vi "ORP电极校准.vi"() -> ()   [LabVIEW 2016, in "斯坦道多参数.lvlib"]
uses:
  <vilib>/Utility/miscctls.llb/LVPointTypeDef.ctl
  <vilib>/Analysis/NI_AALBase.lvlib
  <vilib>/Utility/config.llb/NI_LVConfig.lvlib
panel:
  out "滤波设定":dbl
  in  "刷新按钮":bool
  out "第二点信号值":dbl
  out "第一点信号值":dbl
  out "通讯状态":string
  out "温度":dbl format="%#.2f"
  out "当前信号值":dbl caption="信号值" format="%#.2f"
  in  "校准停止":bool
  in  "校准启动":bool
  out "波形图表":sgl(graph) caption="历史曲线"
  out "第二点校准值":dbl
  out "第一点校准值":dbl
  in  "校准模式":u16(ring) items=["单点校准"]
  out "提示":string
  out "最小值":sgl format="%#.2f"
  out "最大值":sgl format="%#.2f"
  out "mean":dbl caption="均值" format="%#.2f"
  out "standard deviation":dbl caption="标准差" format="%#.2f"
  out "变异系数":dbl format="%#.6f"
  in  "标液1":dbl
  out "当前读取值":dbl caption="测量值" format="%#.2f"
  out "ORP偏移修正值":dbl format="%#.2f"
  # "ORP电极设定"
  # "请选择校准模式:"
  # "℃"
  # "mV"
  # "mV"
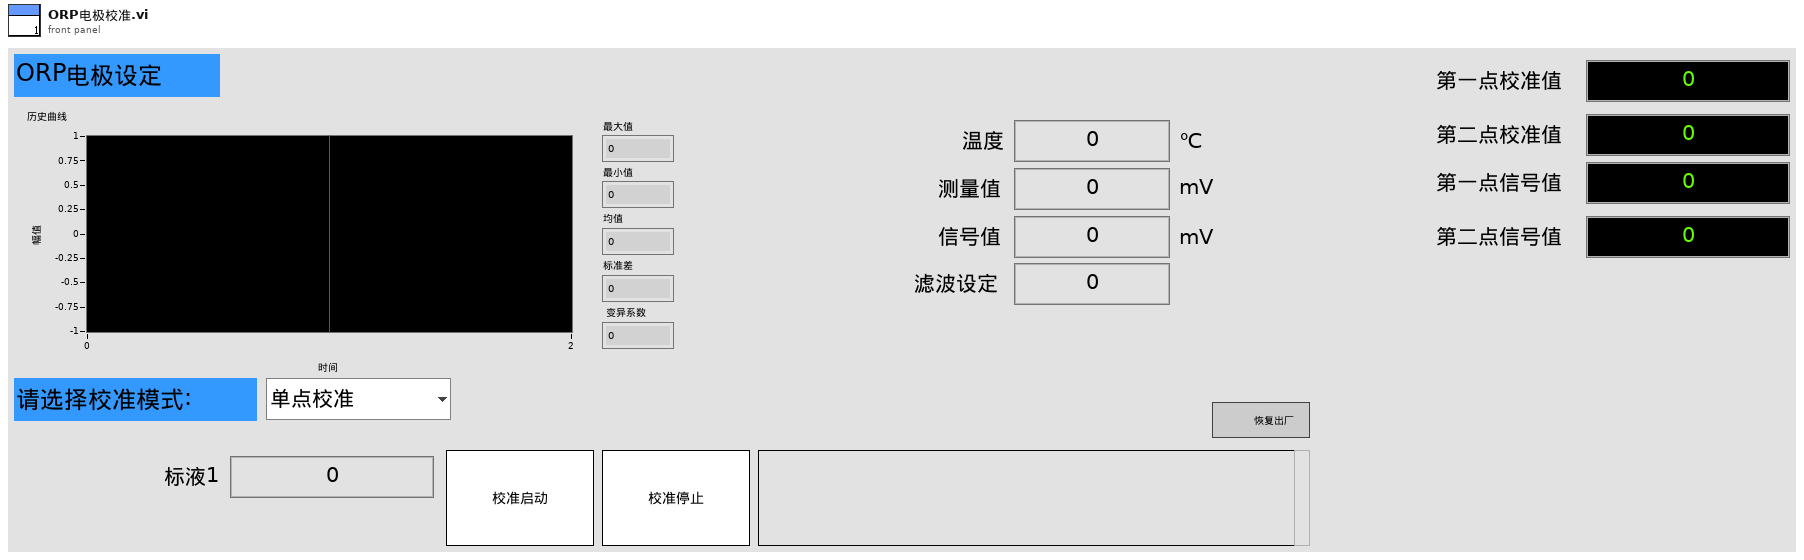
[diagram p1: front panel]
types:
  T1 = typedef "LVPointTypeDef.ctl" = cluster{"Horizontal":i16, "Vertical":i16}
  T2 = typedef "NI_LVConfig.lvlib/Config Data RefNum.ctl" = refnum<k1>
  T3 = cluster{"电极状态标志":u16, "电极型号标志":u16, "测量值":sgl, "温度测量值":sgl, "信号值":sgl, "温度信号值":sgl, "000AH_NC":sgl, "偏移修正值":sgl, "温度偏移修正值":sgl, "手动温度补偿值":sgl, "命令滤波设定":u16, "温度模式":enum16{"ATC", "MTC"}, "生产批次":u16, "传感器序号":u16, "串口地址":u16, "串口波特率":enum16{"9600", "19200", "115200"}, "串口校验位":enum16{"NONE", "ODD", "EVEN"}, "串口停止位":enum16{"1bit", "2bit"}}
  T4 = enum8{"Enabled", "Disabled", "Disabled and Grayed Out"}
  T5 = cluster{"ph":bool, "DO":bool, "Cond":bool, "Turb":bool, "叶绿素a":bool, "藻密度":bool, "ORP":bool}
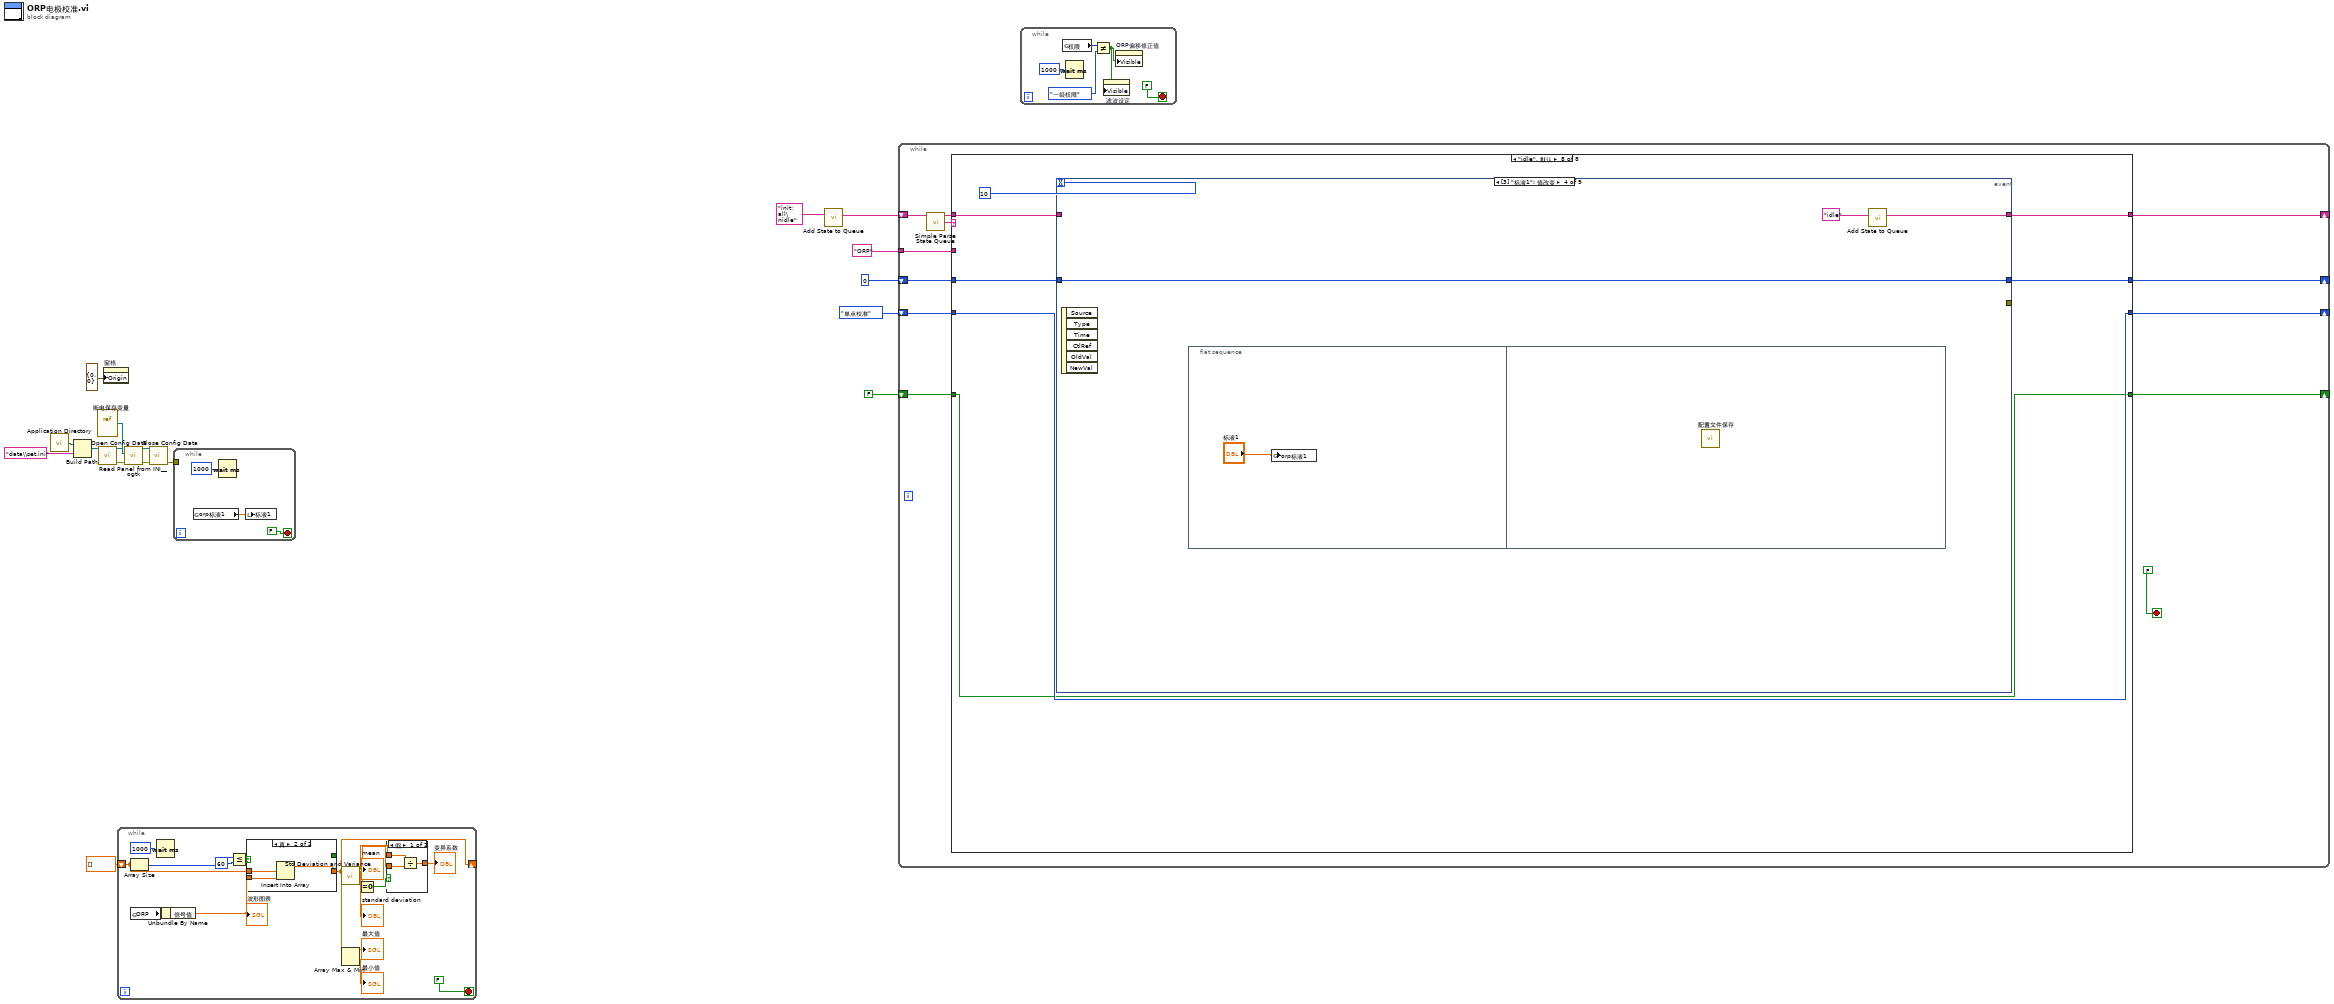
[diagram p0: block diagram]
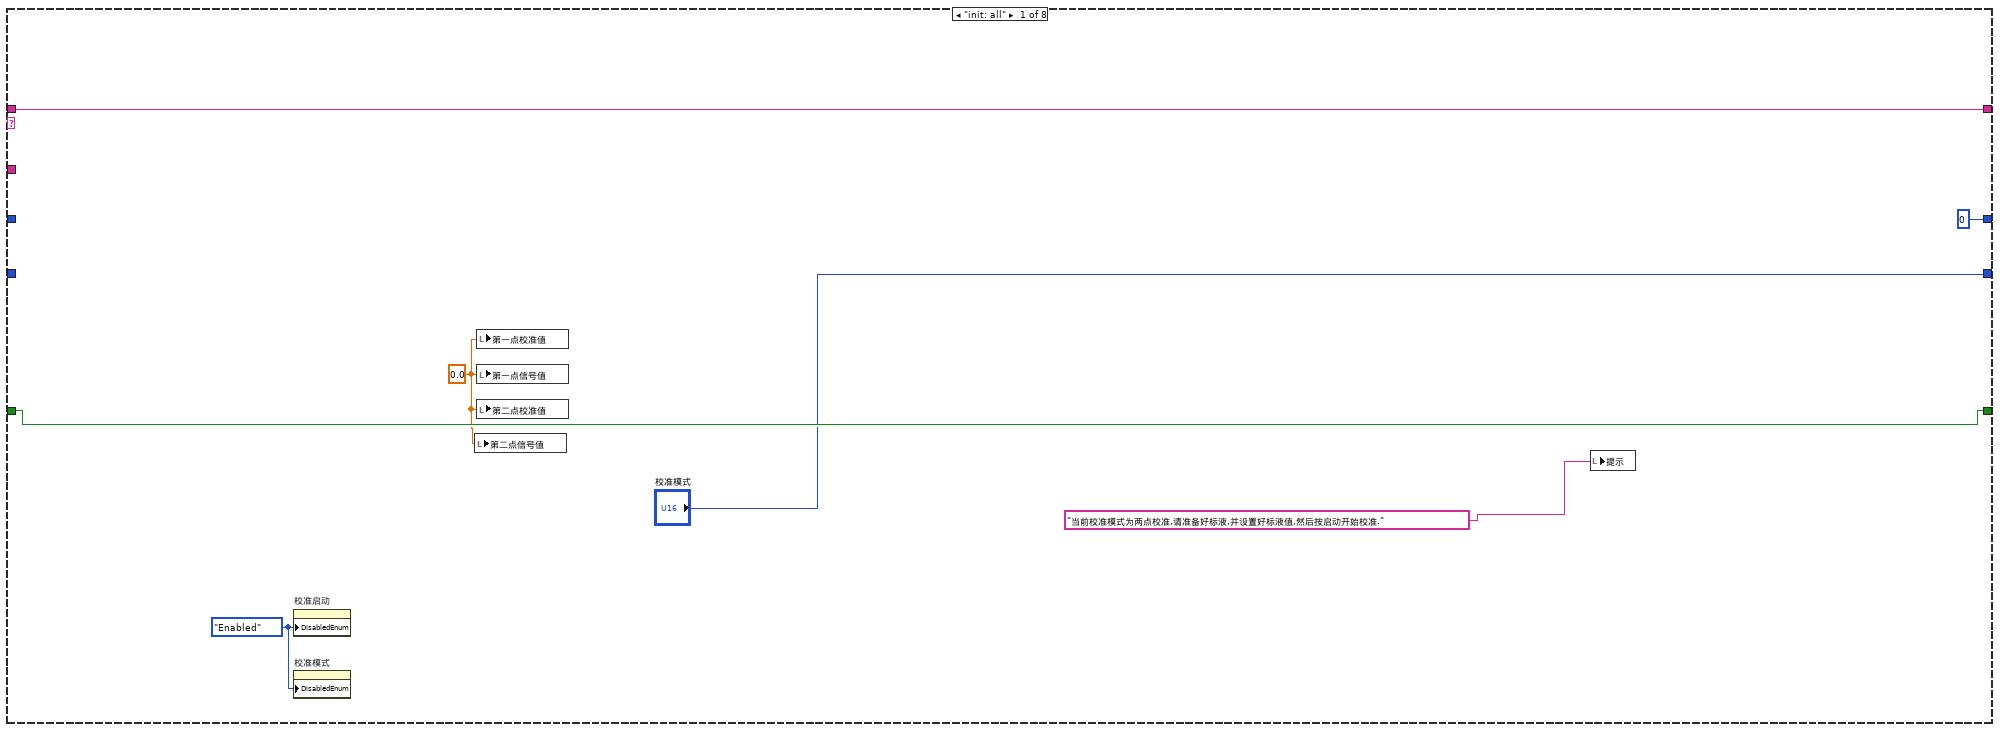
[diagram p2: hidden frame]
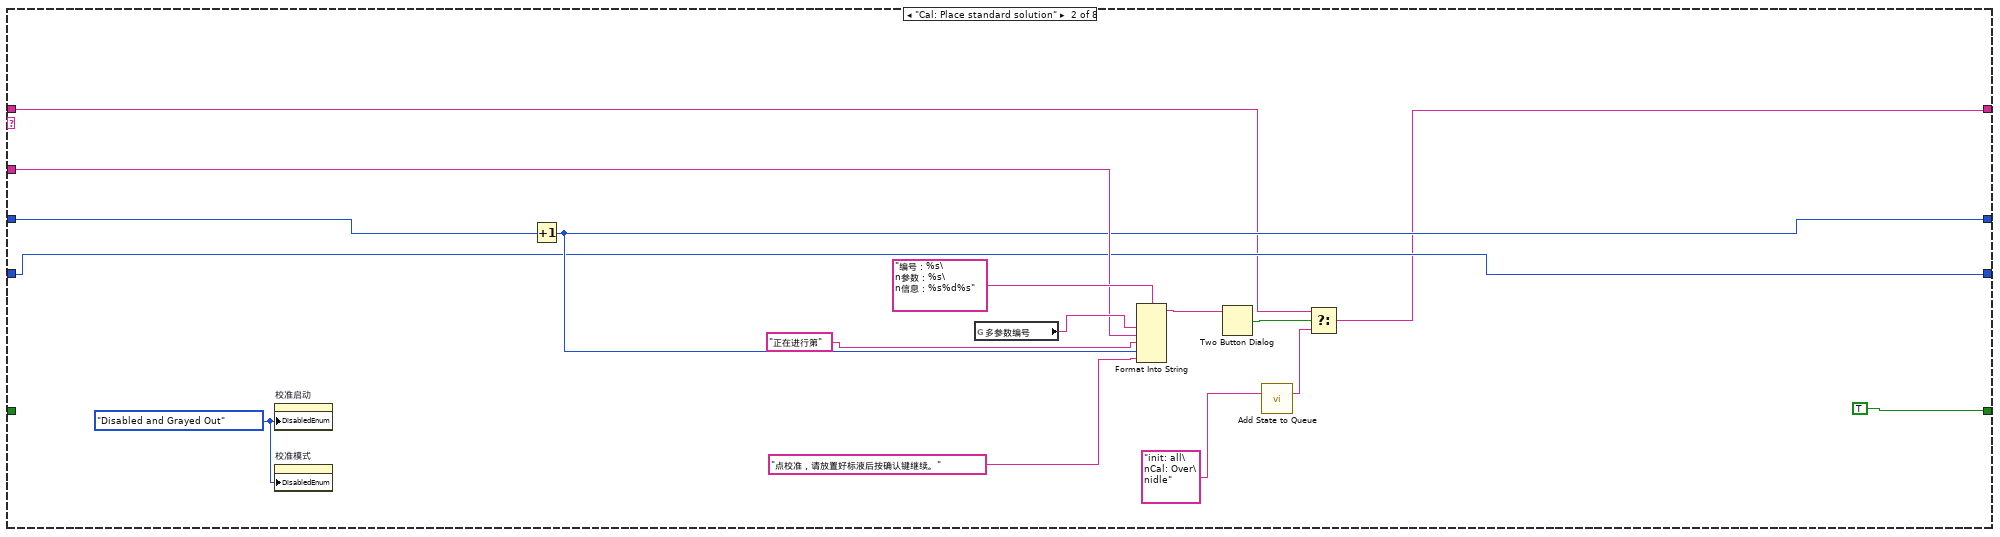
[diagram p3: hidden frame]
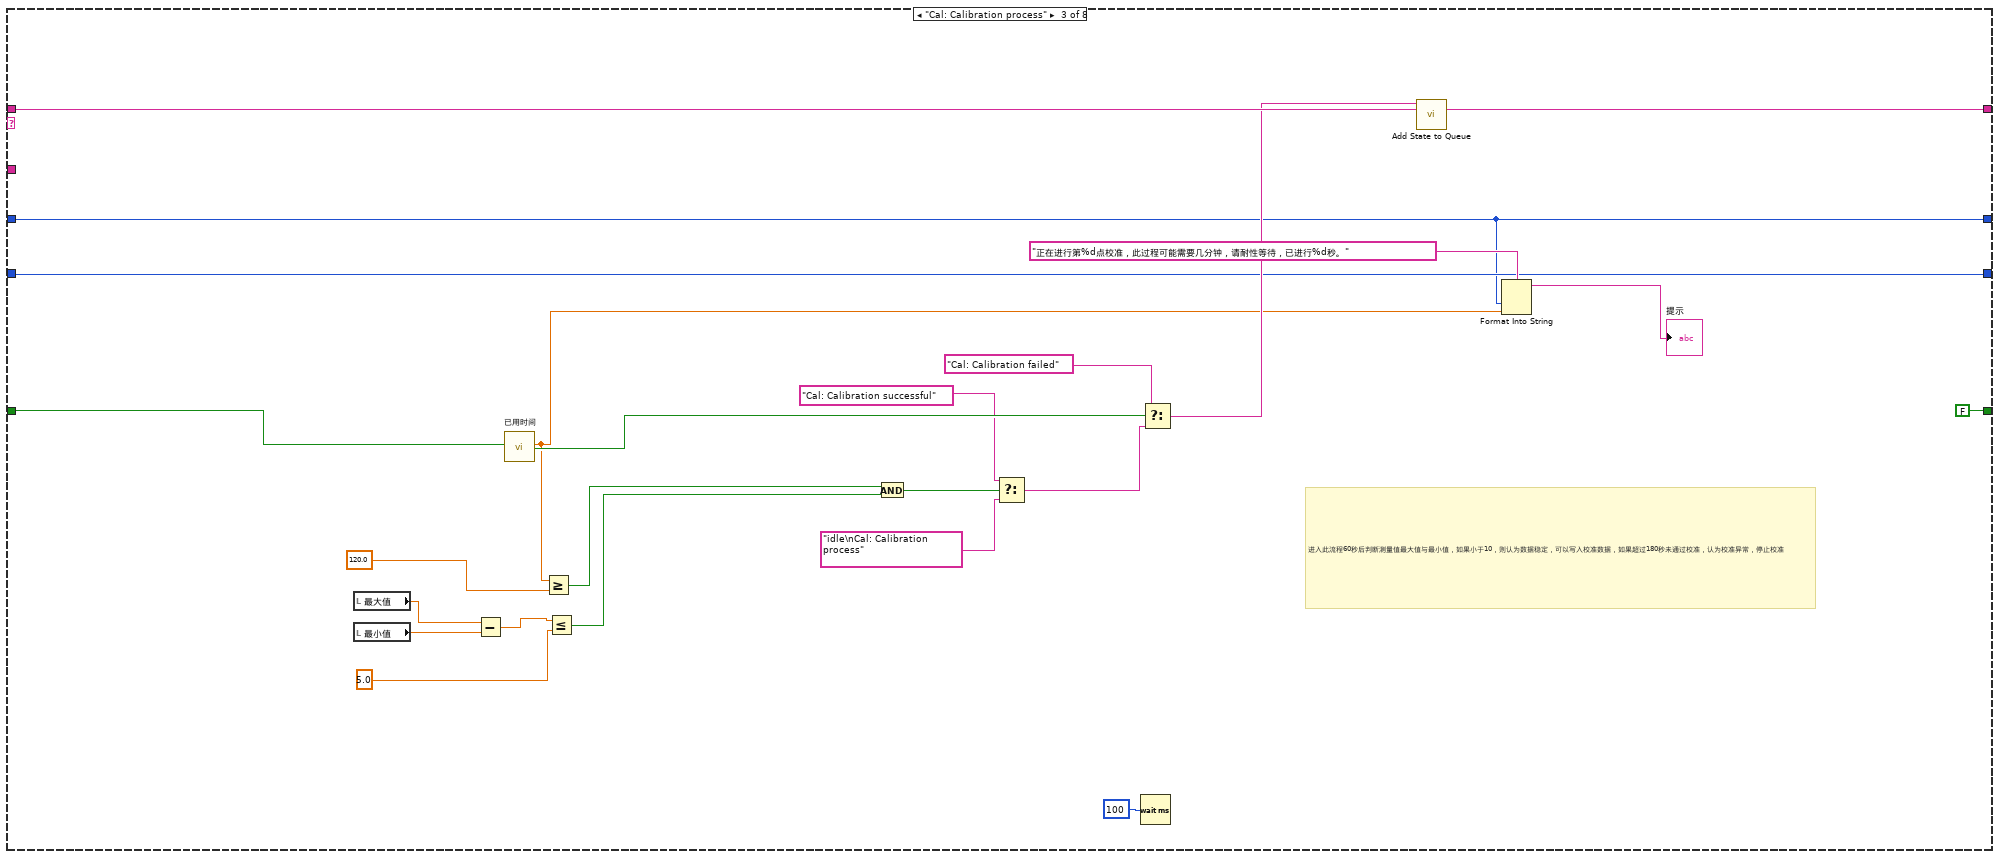
[diagram p4: hidden frame]
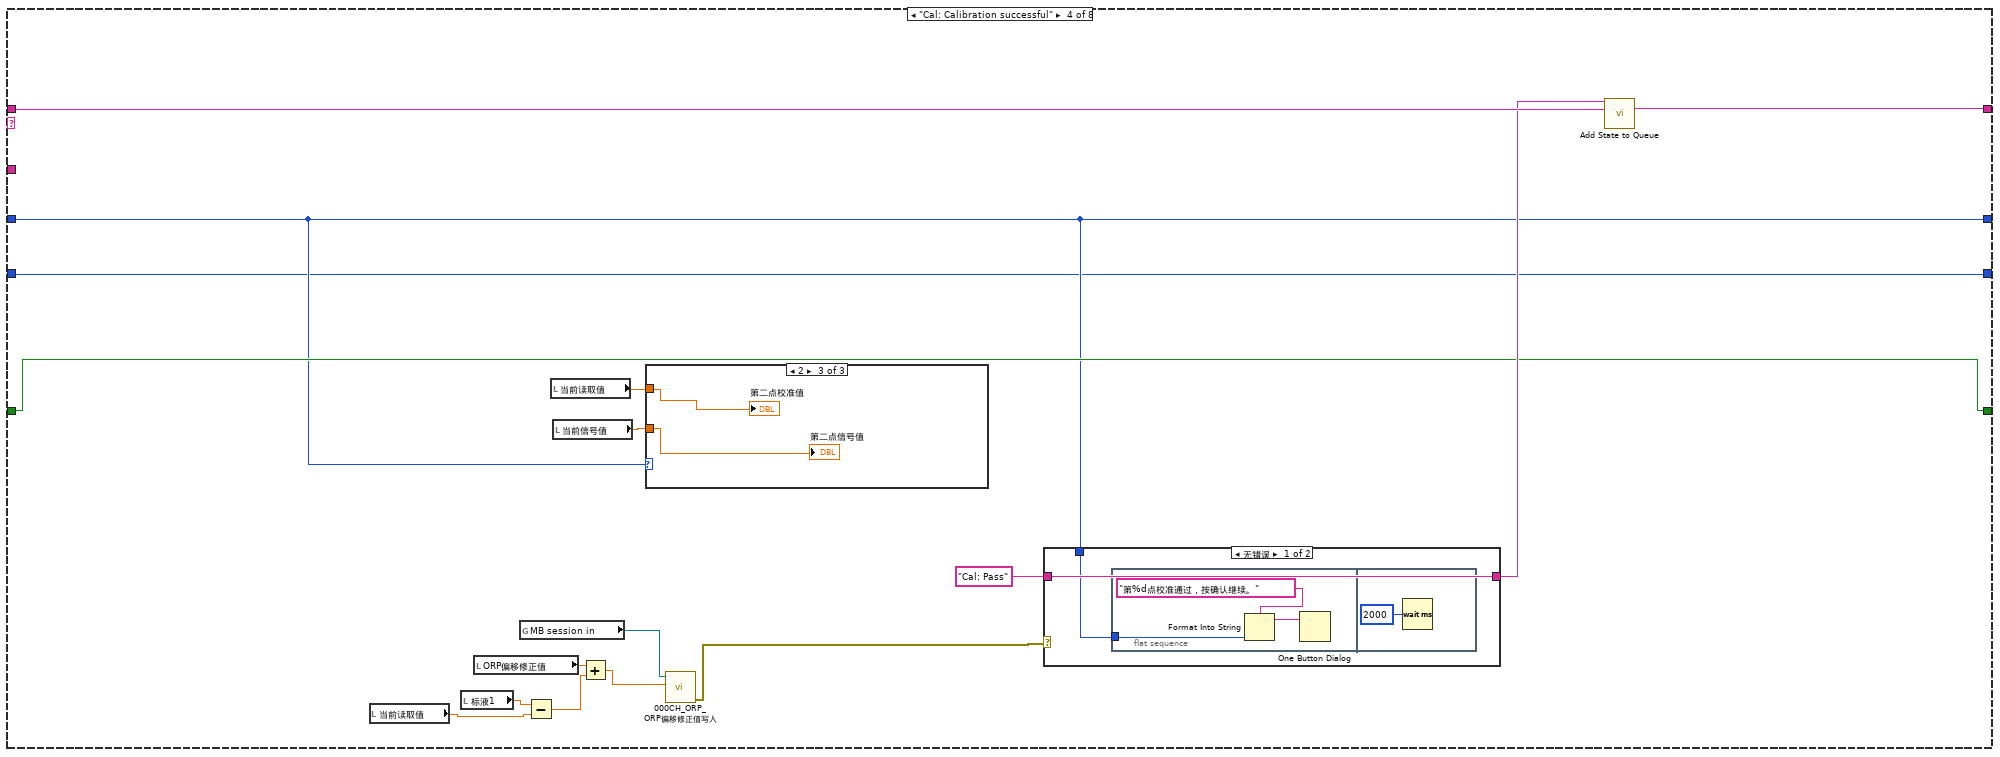
[diagram p5: hidden frame]
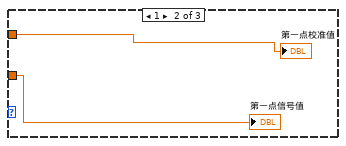
[diagram p7: hidden frame]
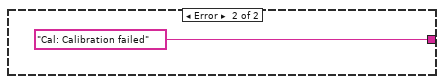
[diagram p8: hidden frame]
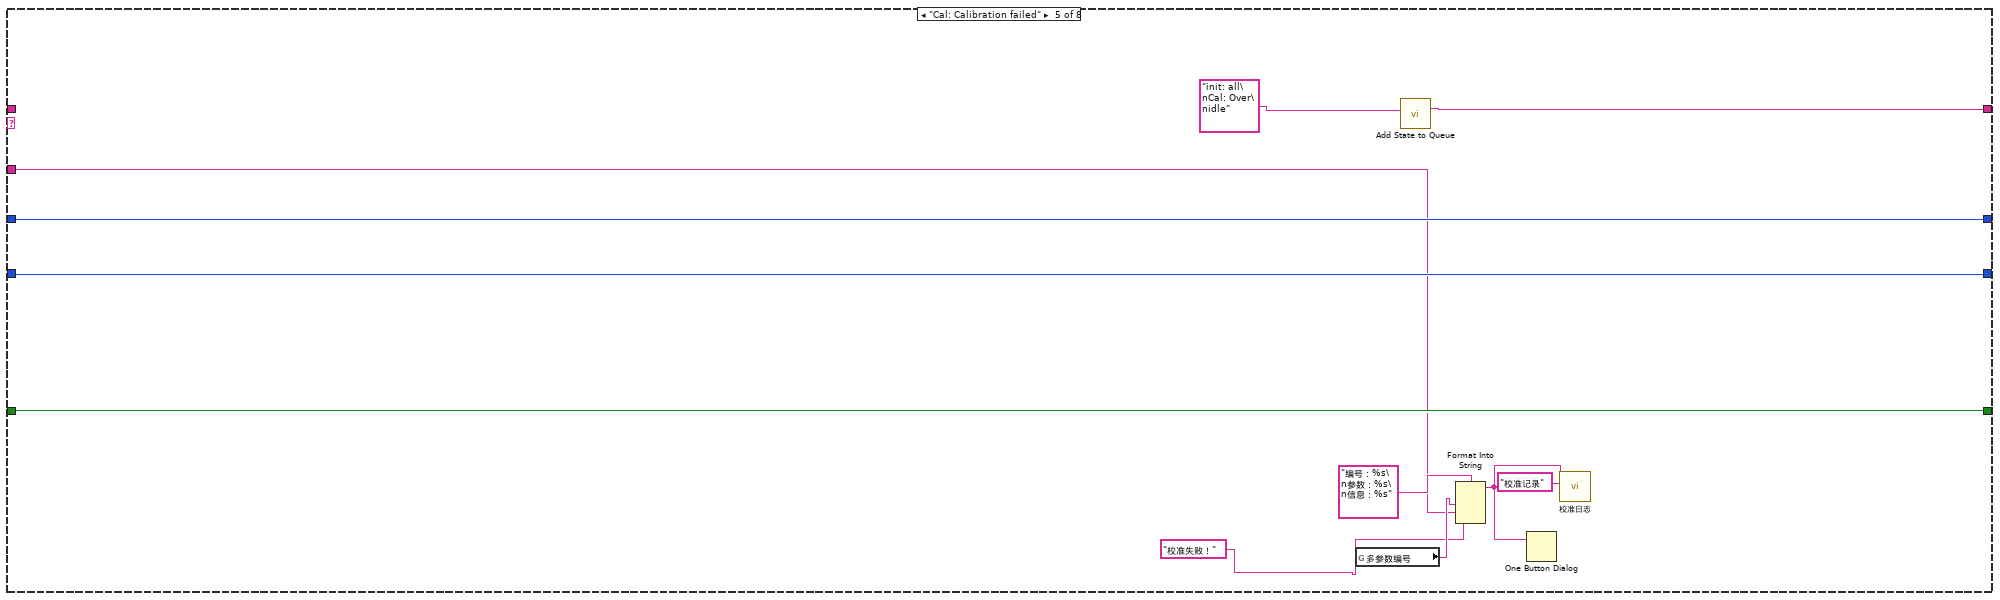
[diagram p9: hidden frame]
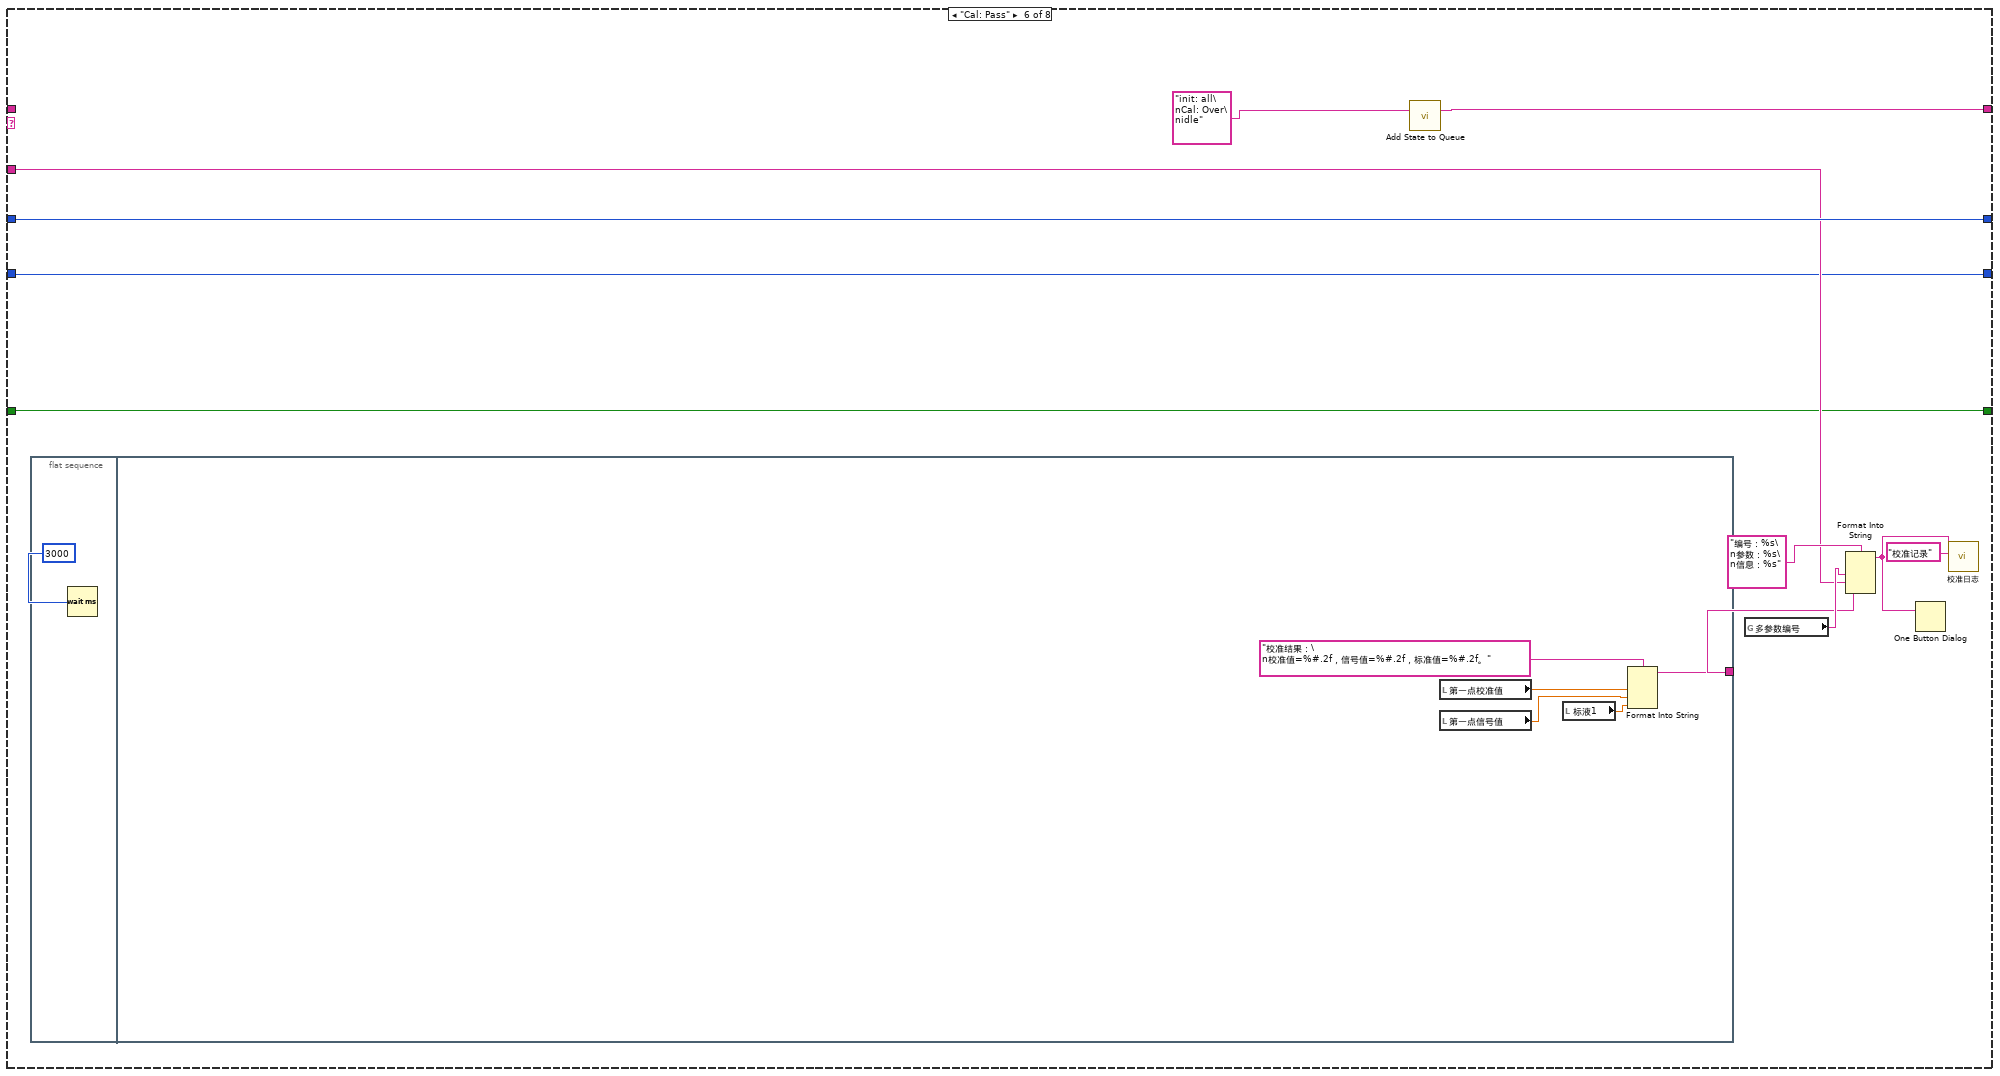
[diagram p10: hidden frame]
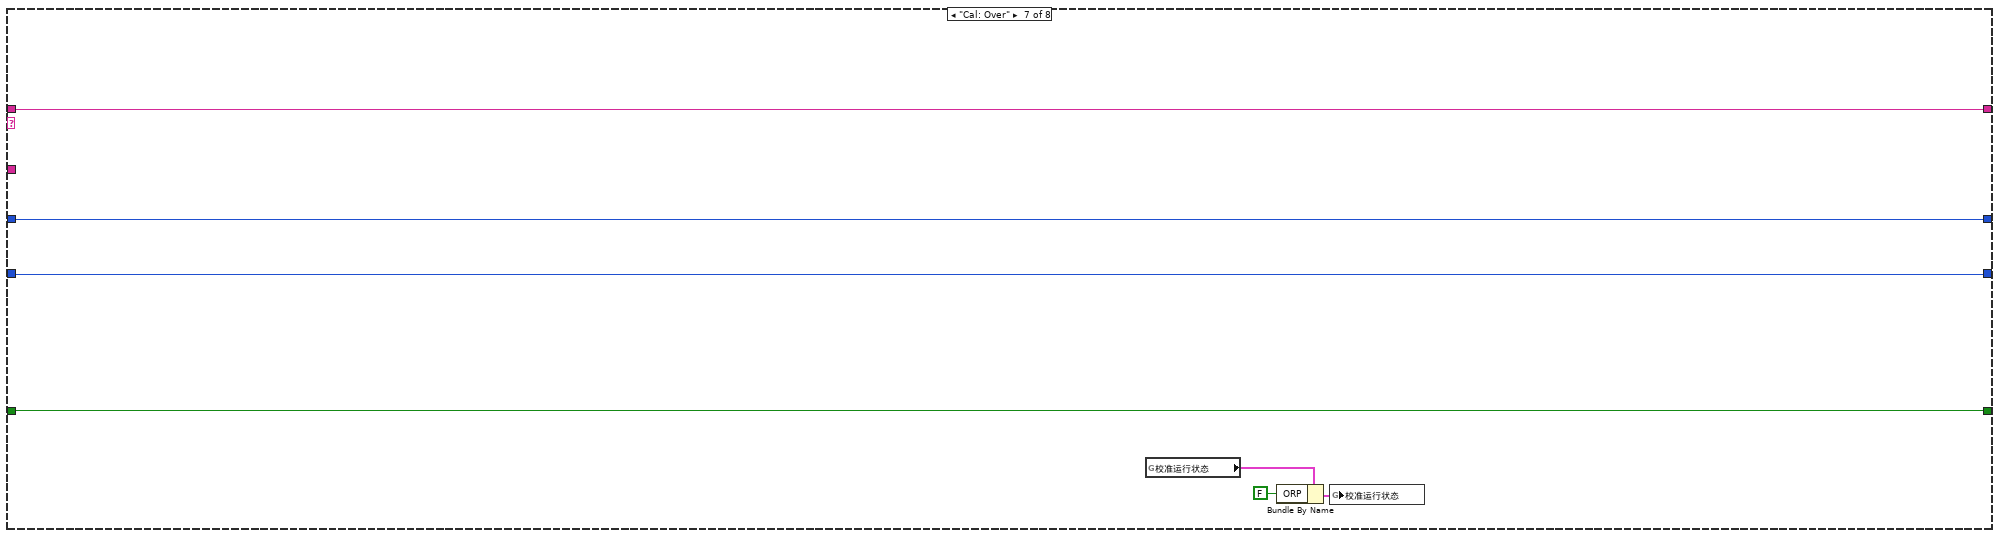
[diagram p11: hidden frame]
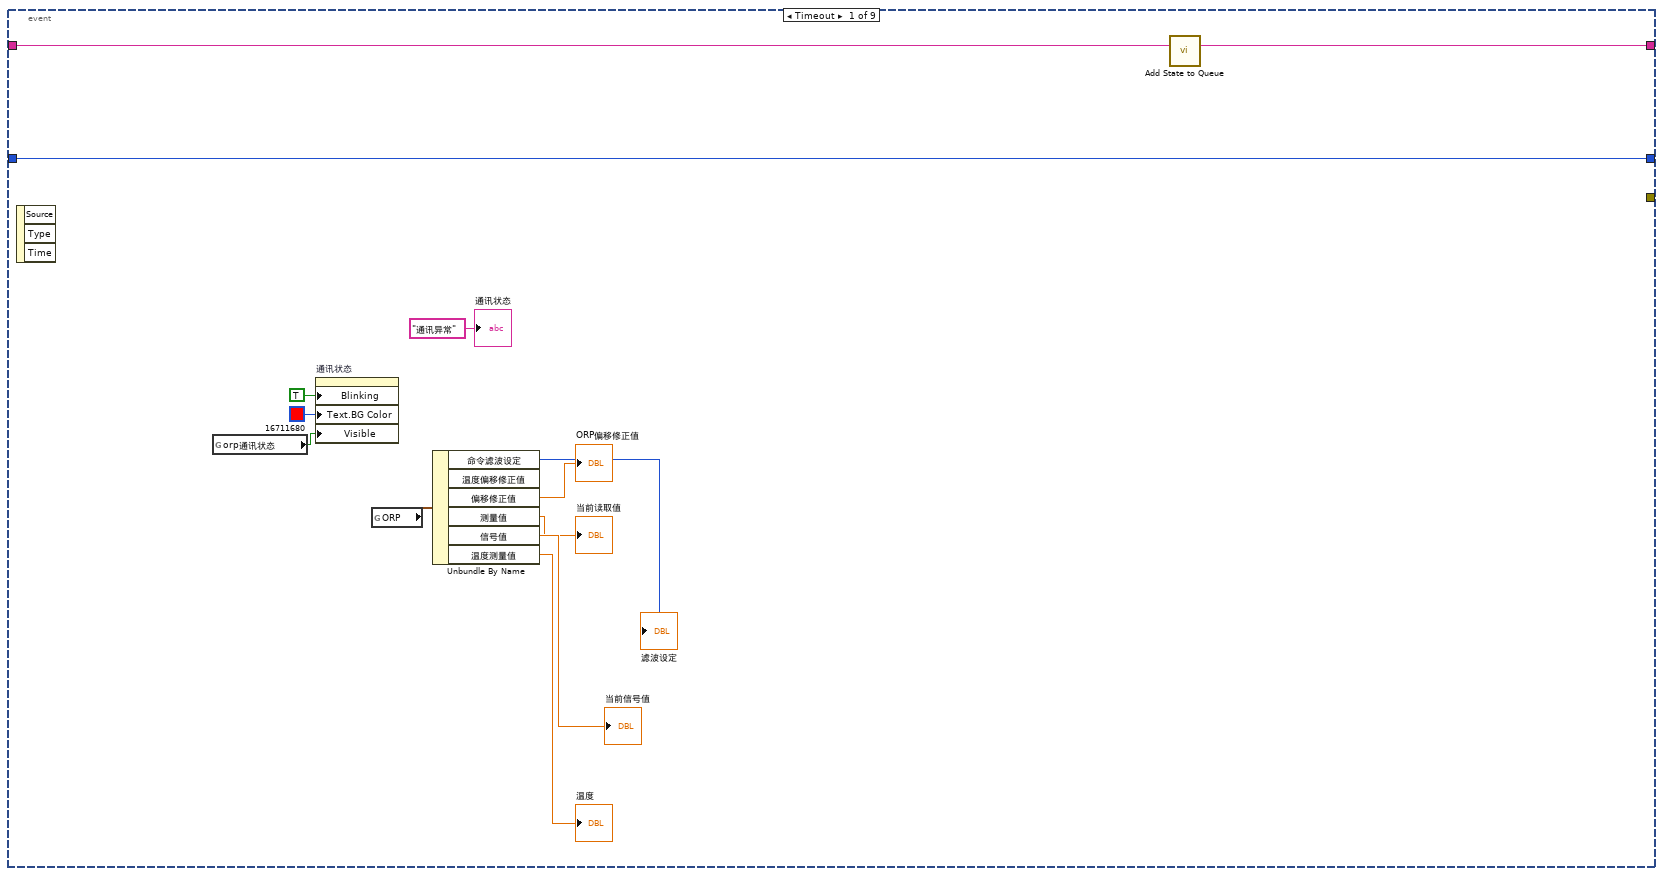
[diagram p12: hidden frame]
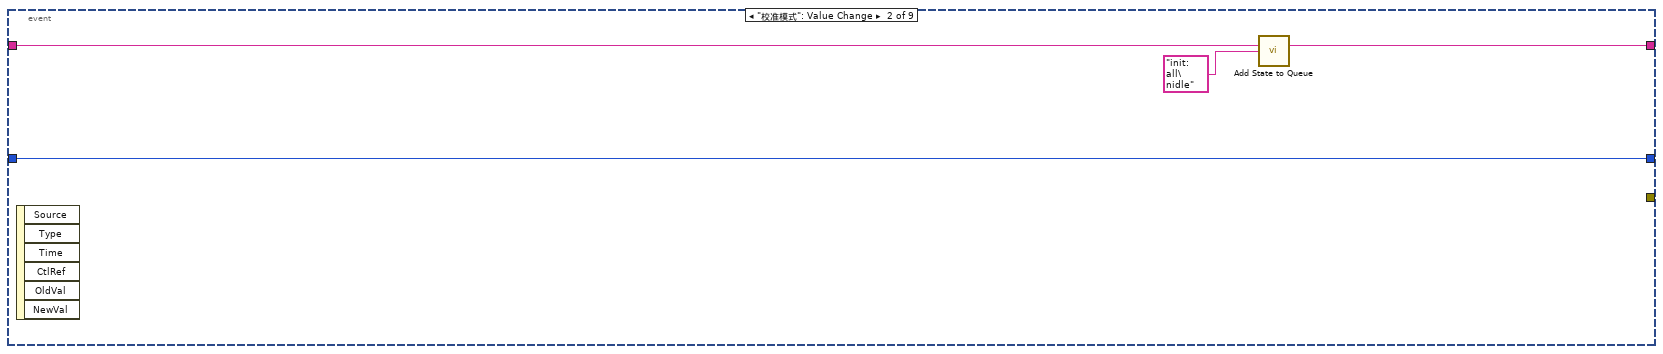
[diagram p13: hidden frame]
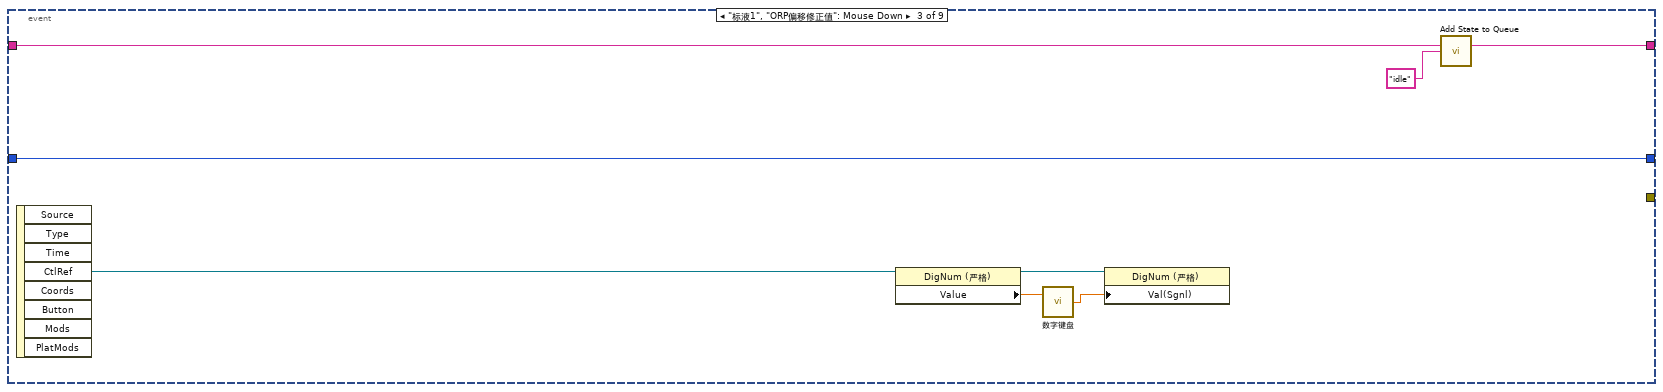
[diagram p14: hidden frame]
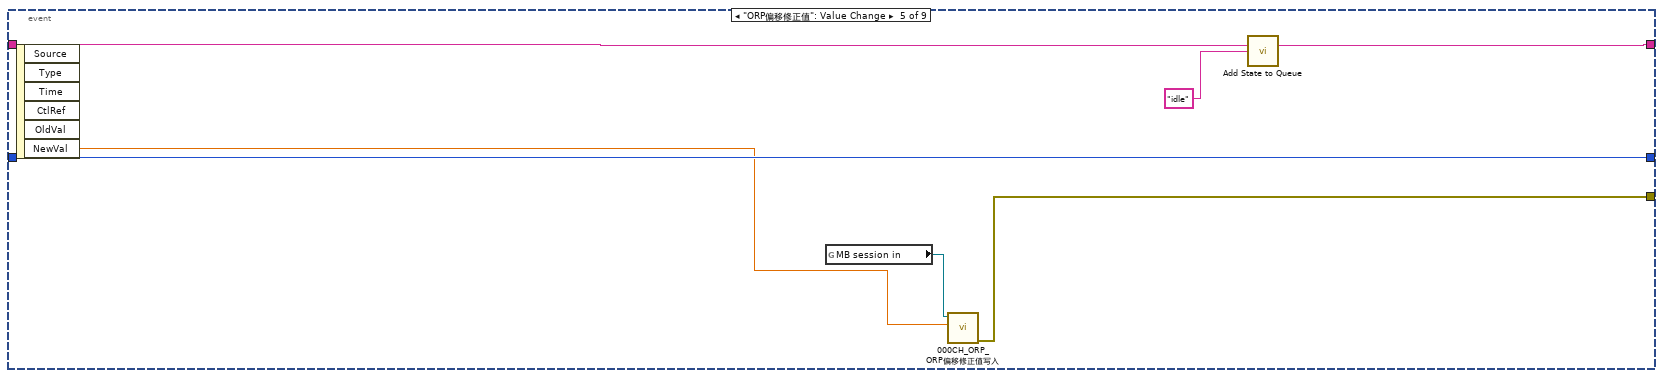
[diagram p15: hidden frame]
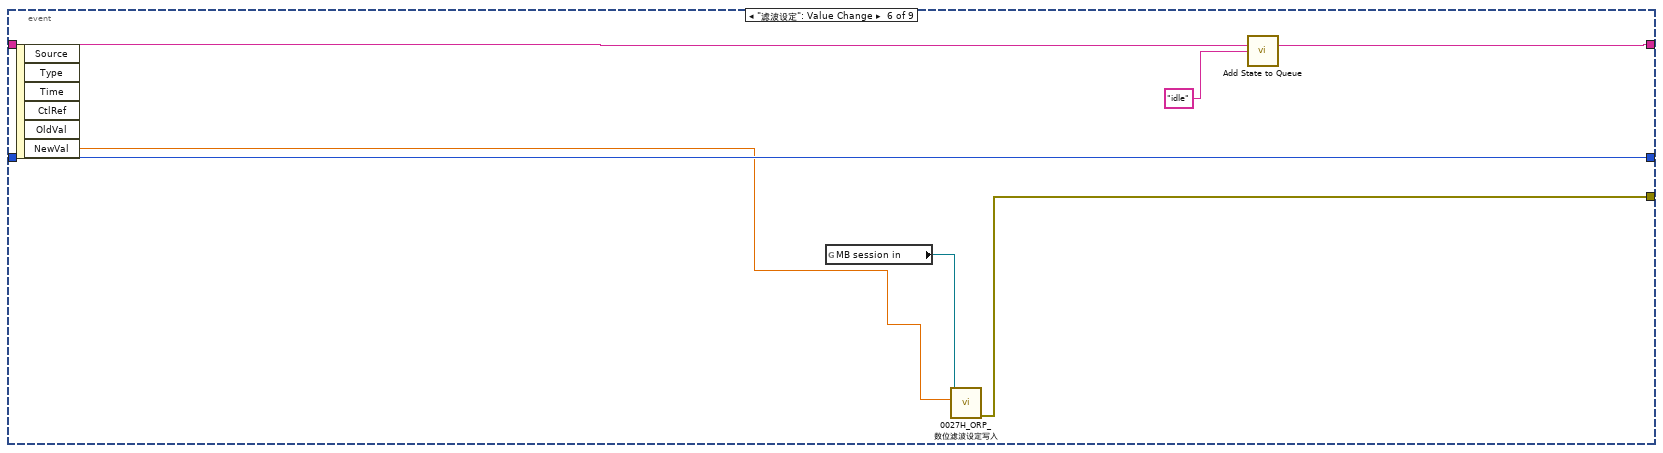
[diagram p16: hidden frame]
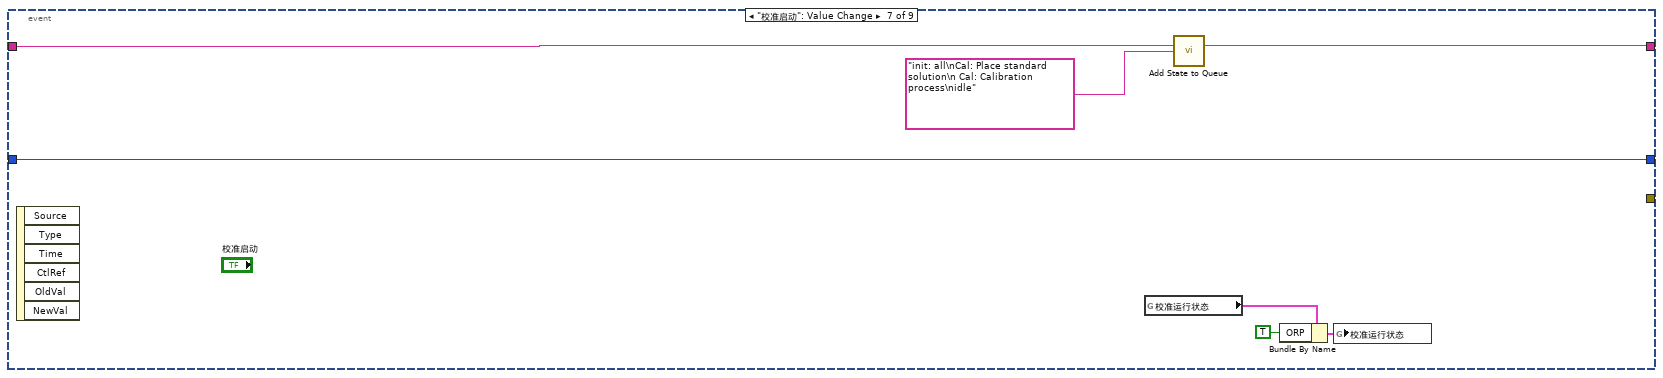
[diagram p17: hidden frame]
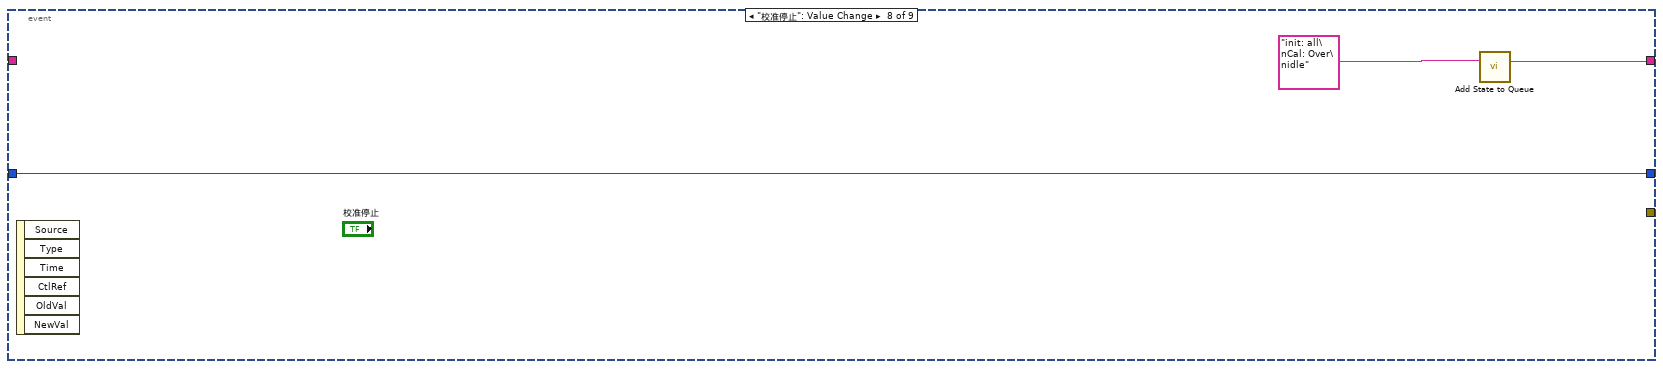
[diagram p18: hidden frame]
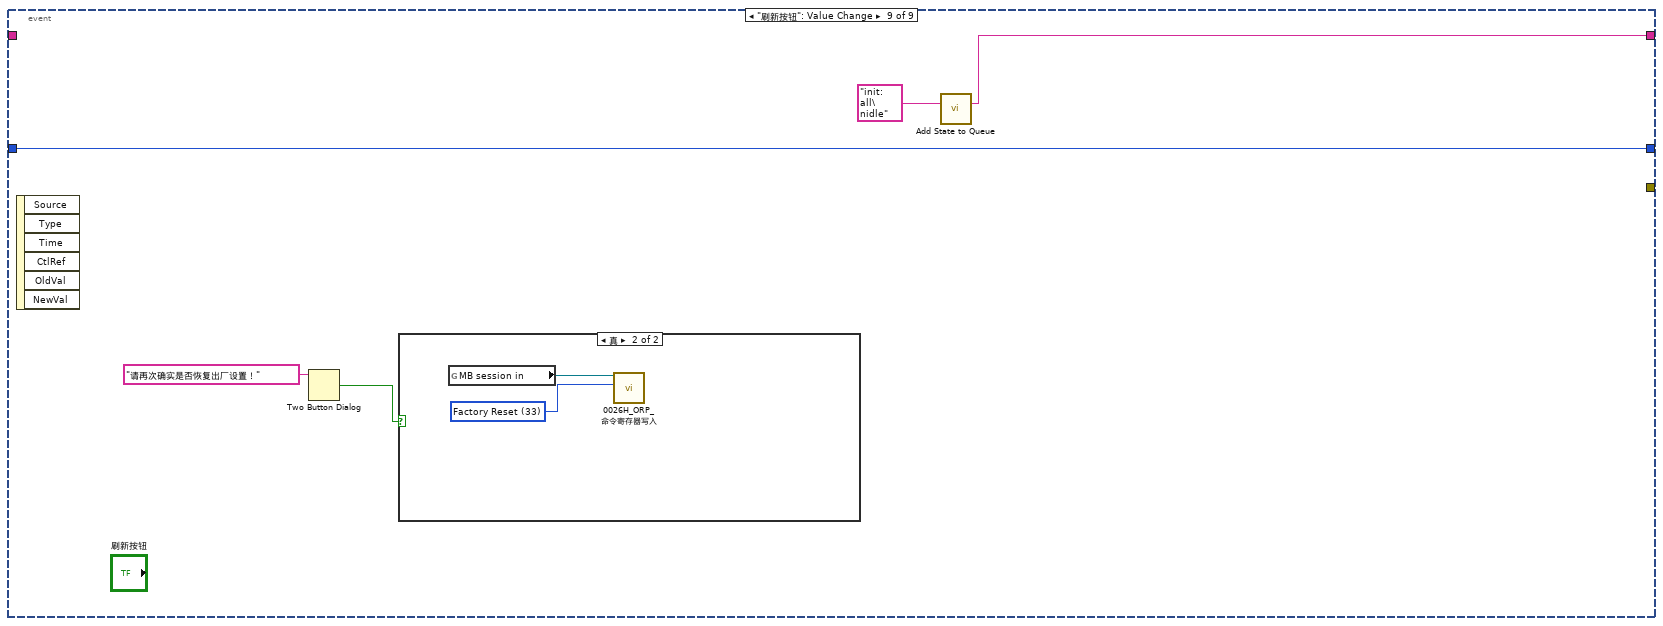
[diagram p19: hidden frame]
diagram:
  n1 = call <vilib>:"Application Directory.vi"() -> ("Application Directory"=w6:path)
  n2 = Build Path(base path=w6, name or relative path="data\\set.ini" ("名称或相对路径")) -> (appended path=w7:path)
  n3 = vi-ref "断电保存变量.vi"() -> (w9:refnum<vi>)
  n4 = call <vilib>:"Open Config Data.vi"("configuration file path"=w7) -> ("error out"=w3:errorcluster, "refnum"=w2:T2)  [unwired: 8 in, 1 out]
  n5 = property on="窗格" class="Pane"("Origin"=T1 {"Horizontal"=0, "Vertical"=0} ("原点")) -> ()  [unwired: 2 in, 2 out]
  n6 = while {
    shift-right: [w21] -> _
    shift-left: sgl[] [] -> [w28]
    stop <- FALSE stop-if-true
    n7 = Array Size(array=w28) -> (size(s)=w30:i32)
    n8 = global read "国弘过程全局变量.vi" "ORP"() -> (w22:T3)
    n9 = Wait (ms)(milliseconds to wait=u32 1000 ("等待时间（毫秒）")) -> ()  [unwired: 1 out]
    n10 = Unbundle By Name(w22) -> ("信号值"=w18:sgl)
    "波形图表" <- w18
    n11 = Less Or Equal?(x=w30, y=60) -> (x <= y?=w29:bool)
    n12 = case shown="真" w29 {
      tunnel: w28 -> [w41 w44]
      tunnel: w18 -> [w39 w43]
      tunnel: [w37 w42] -> w21
      tunnel: [TRUE _] -> _
      frame False {
        n13 = Replace Array Subset(array=w41, new element=w39) -> (w40:sgl[])  [unwired: 1 in]
        n14 = Rotate 1D Array(1:w40, 2:-1 ("n")) -> (0:w37:sgl[])
      }
      frame True {
        n15 = Insert Into Array(array=w44, new element=w43) -> (w42:sgl[])  [unwired: 1 in]
      }
    }
    n16 = call <vilib>:"Std Deviation and Variance.vi"("X"=w21) -> ("mean"=w26:dbl, "standard deviation"=w25:dbl)  [unwired: 1 in, 1 out]
    "mean" <- w26
    "standard deviation" <- w25
    n17 = Array Max & Min(array=w21) -> (max value=→"最大值":sgl, min value=→"最小值":sgl)  [unwired: 2 out]
    n18 = Equal To 0?(x=w26) -> (x = 0?=w27:bool)
    n19 = case shown="假" w27 {
      tunnel: w25 -> [w35 _]
      tunnel: [w34 _] -> w24
      tunnel: w26 -> [w33 _]
      frame False {
        n20 = Divide(x=w35, y=w33) -> (x/y=w34:dbl)
      }
      frame True {
      }
    }
    "变异系数" <- w24
  }
  n21 = call <userlib>:"Read Panel from INI__ogtk.vi"("error in (no error)"=w3, "VI ref"=w9, "refnum"=w2) -> ("error out"=w5:errorcluster, "refnum out"=w4:T2)  [unwired: 7 in]
  n22 = call <vilib>:"Close Config Data.vi"("error in (no error)"=w5, "refnum"=w4) -> ("error out"=w1:errorcluster)  [unwired: 8 in, 1 out]
  n23 = while {
    tunnel: w1 -> [_]
    stop <- FALSE stop-if-true
    n24 = global read "断电保存变量.vi" "orp标液1"() -> (w45:dbl)
    n25 = Wait (ms)(milliseconds to wait=u32 1000 ("等待时间（毫秒）")) -> ()  [unwired: 1 out]
    n26 = local write "标液1"(w45) -> ()
  }
  n27 = call "Add State to Queue.vi"("State(s) In (\"\")"="init: all\nidle" ("State(s) In (\"\")")) -> ("States Out"=w14:string)  [unwired: 14 in]
  n28 = while {
    shift-right: [w55] -> _
    shift-left: w14 -> [w59]
    shift-right: [w52] -> _
    shift-left: 0 -> [w54]
    tunnel: "ORP" ("State(s) In (\"\")") -> [w53]
    shift-right: [w50] -> _
    shift-left: enum16{"单点校准"}."单点校准" ("校准模式") -> [w51]
    shift-right: [w48] -> _
    shift-left: FALSE -> [w49]
    stop <- FALSE stop-if-true
    n29 = call "Simple Parse State Queue.vi"("State Queue"=w59) -> ("Remain States"=w56:string, "Next State"=w57:string)  [unwired: 13 in]
    n30 = case shown="\"idle\", 默认" w57 {
      tunnel: w56 -> [w66 w70 w101 w121 _ _ w165 w175]
      tunnel: [w66 w69 w100 w120 w141 w146 w165 w174] -> w55
      tunnel: w54 -> [_ w78 w85 w115 w144 w155 w162 w172]
      tunnel: w53 -> [_ w79 _ _ w135 w151 _ _]
      tunnel: [0 w76 w85 w115 w144 w155 w162 w173] -> w52
      tunnel: w51 -> [_ w75 w86 w114 w143 w147 w163 w171]
      tunnel: ["校准模式" w75 w86 w114 w143 w147 w163 w171] -> w50
      tunnel: w49 -> [w63 _ w88 w116 w142 w150 w164 w169]
      tunnel: [w63 TRUE FALSE w116 w142 w150 w164 w169] -> w48
      frame "init: all" {
        w61 = T4."Enabled" ("禁用")
        w60 = 0.0 ("第一点校准值")
        n31 = property on="校准启动" class="Bool"("DisabledEnum"=w61) -> ()  [unwired: 2 in, 2 out]
        n32 = property on="校准模式" class="Ring (严格)"("DisabledEnum"=w61) -> ()  [unwired: 2 in, 2 out]
        n33 = local write "第二点信号值"(w60) -> ()
        n34 = local write "第一点校准值"(w60) -> ()
        n35 = local write "第一点信号值"(w60) -> ()
        n36 = local write "第二点校准值"(w60) -> ()
        n37 = local write "提示"("当前校准模式为两点校准,请准备好标液,并设置好标液值,然后按启动开始校准." ("提示")) -> ()
      }
      frame "Cal: Place standard solution" {
        w68 = T4."Disabled and Grayed Out" ("禁用")
        n38 = property on="校准启动" class="Bool"("DisabledEnum"=w68) -> ()  [unwired: 2 in, 2 out]
        n39 = property on="校准模式" class="Ring (严格)"("DisabledEnum"=w68) -> ()  [unwired: 2 in, 2 out]
        n40 = Increment(x=w78) -> (x+1=w76:i32)
        n41 = global read "多参数全局变量.vi" "多参数编号"() -> (w81:string)
        n42 = Format Into String(format string="编号：%s\n参数：%s\n信息：%s%d%s" ("格式字符串"), w81, w79, "正在进行第" ("消息"), w76, "点校准，请放置好标液后按确认键继续。" ("消息")) -> (resulting string=w73:string)  [unwired: 2 in, 1 out]
        n43 = Two Button Dialog(message=w73) -> (T button?=w72:bool)  [unwired: 2 in]
        n44 = call "Add State to Queue.vi"("State(s) In (\"\")"="init: all\nCal: Over\nidle" ("State(s) In (\"\")")) -> ("States Out"=w71:string)  [unwired: 14 in]
        n45 = Select(t=w70, s=w72, f=w71) -> (s? t:f=w69:string)
      }
      frame "Cal: Calibration process" {
        # "进入此流程60秒后判断测量值最大值与最小值，如果小于10，则认为数据稳定，可以写入校准数据，如果超过180秒未通过校准，认为校准异常，停止校准"
        n46 = local read "最大值"() -> (w105:sgl)
        n47 = local read "最小值"() -> (w104:sgl)
        n48 = Subtract(x=w105, y=w104) -> (x-y=w106:sgl)
        n49 = call "已用时间"("Reset"=w88) -> ("Elapsed Time (s)"=w84:dbl, "Time has Elapsed"=w102:bool)  [unwired: 11 in, 6 out]
        n50 = Greater Or Equal?(x=w84, y=120.0) -> (x >= y?=w97:bool)
        n51 = Less Or Equal?(x=w106, y=5.0) -> (x <= y?=w93:bool)
        n52 = And(x=w97, y=w93) -> (x .and. y?=w94:bool)
        n53 = Select(t="Cal: Calibration successful" ("State(s) In (\"\")"), s=w94, f="idle\nCal: Calibration process" ("State(s) In (\"\")")) -> (s? t:f=w92:string)
        n54 = Wait (ms)(milliseconds to wait=u32 100 ("等待时间（毫秒）")) -> ()  [unwired: 1 out]
        n55 = Select(t="Cal: Calibration failed" ("State(s) In (\"\")"), s=w102, f=w92) -> (s? t:f=w91:string)
        n56 = call "Add State to Queue.vi"("State(s) In Front (\"\")"=w91, "State(s) In (\"\")"=w101) -> ("States Out"=w100:string)  [unwired: 13 in]
        n57 = Format Into String(format string="正在进行第%d点校准，此过程可能需要几分钟，请耐性等待，已进行%d秒。" ("格式字符串"), w85, w84) -> (resulting string=→"提示":string)  [unwired: 2 in, 1 out]
      }
      frame "Cal: Calibration successful" {
        n58 = local read "当前读取值"() -> (w110:dbl)
        n59 = local read "标液1"() -> (w113:dbl)
        n60 = local read "ORP偏移修正值"() -> (w111:dbl)
        n61 = global read "多参数全局变量.vi" "MB session in"() -> (w109:refnum<class "MB_Master.lvclass">)
        n62 = Subtract(x=w113, y=w110) -> (x-y=w112:dbl)
        n63 = local read "当前读取值"() -> (w117:dbl)
        n64 = local read "当前信号值"() -> (w118:dbl)
        n65 = Add(x=w111, y=w112) -> (x+y=w108:dbl)
        n66 = case shown="2" w115 {
          tunnel: w118 -> [_ w124 w126]
          tunnel: w117 -> [_ w123 w125]
          frame 0, Default {
          }
          frame 1 {
            "第一点信号值" <- w124
            "第一点校准值" <- w123
          }
          frame 2 {
            "第二点信号值" <- w126
            "第二点校准值" <- w125
          }
        }
        n67 = call "000CH_ORP_ORP偏移修正值写入.vi"("数值"=w108, "MB session in"=w109) -> ("error out"=w107:errorcluster)  [unwired: 8 in, 1 out]
        n68 = case shown="无错误" w107 {
          tunnel: "Cal: Pass" ("State(s) In (\"\")") -> [w128 _]
          tunnel: [w128 "Cal: Calibration failed" ("State(s) In (\"\")")] -> w119
          tunnel: w115 -> [w127 _]
          frame No Error {
            n69 = flat-sequence {
              tunnel: w127 -> [w129]
              frame #0 {
                n70 = Format Into String(format string="第%d点校准通过，按确认继续。" ("格式字符串"), w129) -> (resulting string=w131:string)  [unwired: 2 in, 1 out]
                n71 = One Button Dialog(message=w131) -> ()  [unwired: 1 in, 1 out]
              }
              frame #1 {
                n72 = Wait (ms)(milliseconds to wait=u32 2000 ("等待时间（毫秒）")) -> ()  [unwired: 1 out]
              }
            }
          }
          frame Error {
          }
        }
        n73 = call "Add State to Queue.vi"("State(s) In Front (\"\")"=w119, "State(s) In (\"\")"=w121) -> ("States Out"=w120:string)  [unwired: 13 in]
      }
      frame "Cal: Calibration failed" {
        n74 = global read "多参数全局变量.vi" "多参数编号"() -> (w138:string)
        n75 = call "Add State to Queue.vi"("State(s) In (\"\")"="init: all\nCal: Over\nidle" ("State(s) In (\"\")")) -> ("States Out"=w141:string)  [unwired: 14 in]
        n76 = Format Into String(format string="编号：%s\n参数：%s\n信息：%s" ("格式字符串"), w138, w135, "校准失败！" ("消息")) -> (resulting string=w137:string)  [unwired: 2 in, 1 out]
        n77 = One Button Dialog(message=w137) -> ()  [unwired: 1 in, 1 out]
        n78 = call "校准日志.vi"("table"="校准记录", "日志信息"=w137) -> ()  [unwired: 9 in, 1 out]
      }
      frame "Cal: Pass" {
        n79 = flat-sequence {
          tunnel: [w161] -> w148
          frame #0 {
            n80 = Wait (ms)(milliseconds to wait=u32 3000 ("等待时间（毫秒）")) -> ()  [unwired: 1 out]
          }
          frame #1 {
            n81 = local read "第一点校准值"() -> (w160:dbl)
            n82 = local read "第一点信号值"() -> (w158:dbl)
            n83 = local read "标液1"() -> (w157:dbl)
            n84 = Format Into String(format string="校准结果：\n校准值=%#.2f，信号值=%#.2f，标准值=%#.2f。" ("提示"), w160, w158, w157) -> (resulting string=w161:string)  [unwired: 2 in, 1 out]
          }
        }
        n85 = call "Add State to Queue.vi"("State(s) In (\"\")"="init: all\nCal: Over\nidle" ("State(s) In (\"\")")) -> ("States Out"=w146:string)  [unwired: 14 in]
        n86 = global read "多参数全局变量.vi" "多参数编号"() -> (w152:string)
        n87 = Format Into String(format string="编号：%s\n参数：%s\n信息：%s" ("格式字符串"), w152, w151, w148) -> (resulting string=w149:string)  [unwired: 2 in, 1 out]
        n88 = One Button Dialog(message=w149) -> ()  [unwired: 1 in, 1 out]
        n89 = call "校准日志.vi"("table"="校准记录", "日志信息"=w149) -> ()  [unwired: 9 in, 1 out]
      }
      frame "Cal: Over" {
        n90 = global read "多参数全局变量.vi" "校准运行状态"() -> (w167:T5)
        n91 = Bundle By Name(cluster=w167, "ORP"=FALSE) -> (w168:T5)
        n92 = global write "多参数全局变量.vi" "校准运行状态"(w168) -> ()
      }
      frame "idle", Default {
        n93 = event shown="[3] \"标液1\": 值改变" {
          selector: _ -> [_ _ _ _ _ _ _ _ _]
          dyn-events: _ -> [_ _ _ _ _ _ _ _ _]
          timeout: 10 -> [_ _ _ _ _ _ _ _ _]
          tunnel: [_ _ _ _ w206 w212 _ _ _] -> _
          tunnel: w175 -> [w188 w192 w197 _ w211 w218 w225 _ _]
          tunnel: [w187 w191 w199 w201 w210 w217 w224 w227 w230] -> w174
          tunnel: [w186 w189 w200 w203 w209 w216 w222 w228 w229] -> w173
          tunnel: w172 -> [w186 w189 w200 w203 w209 w216 w222 w228 w229]
          event Timeout {
            n94 = event-data() -> ()  [unwired: 1 in, 3 out]
            n95 = global read "多参数全局变量.vi" "orp通讯状态"() -> (w184:bool)
            n96 = property on="通讯状态" class="Str"("Blinking"=TRUE ("闪烁"), "Text.BG Color"=u32 16711680, "Visible"=w184) -> ()  [unwired: 2 in, 2 out]
            n97 = global read "国弘过程全局变量.vi" "ORP"() -> (w177:T3)
            n98 = Unbundle By Name(w177) -> ("命令滤波设定"=→"滤波设定":u16, "偏移修正值"=→"ORP偏移修正值":sgl, "测量值"=→"当前读取值":sgl, "信号值"=→"当前信号值":sgl, "温度测量值"=→"温度":sgl)  [unwired: 1 out]
            n99 = call "Add State to Queue.vi"("State(s) In (\"\")"=w188) -> ("States Out"=w187:string)  [unwired: 14 in]
            "通讯状态" <- "通讯异常" ("当前串口")
          }
          event "校准模式": Value Change {
            n100 = event-data() -> ()  [unwired: 1 in, 6 out]
            n101 = call "Add State to Queue.vi"("State(s) In (\"\")"=w192, "State(s) At Back (\"\")"="init: all\nidle" ("State(s) In (\"\")")) -> ("States Out"=w191:string)  [unwired: 13 in]
          }
          event "标液1", "ORP偏移修正值": Mouse Down {
            n102 = event-data() -> ("CtlRef"=w196:refnum<vi>)  [unwired: 1 in, 7 out]
            n103 = property class="DigNum (严格)"(reference=w196) -> (reference out=w193:refnum<vi>, "Value"=w194:dbl)  [unwired: 1 in, 1 out]
            n104 = call "数字键盘.vi"("OldNumber"=w194) -> ("NewNumber"=w195:dbl)  [unwired: 1 in]
            n105 = property class="DigNum (严格)"(reference=w193, "Val(Sgnl)"=w195) -> ()  [unwired: 1 in, 2 out]
            n106 = call "Add State to Queue.vi"("State(s) In (\"\")"=w197, "State(s) At Back (\"\")"="idle" ("State(s) In (\"\")")) -> ("States Out"=w199:string)  [unwired: 13 in]
          }
          event "标液1": Value Change {
            n107 = event-data() -> ()  [unwired: 1 in, 6 out]
            n108 = flat-sequence {
              frame #0 {
                n109 = global write "断电保存变量.vi" "orp标液1"("标液1") -> ()
              }
              frame #1 {
                n110 = call "配置文件保存.vi"() -> ()  [unwired: 12 in]
              }
            }
            n111 = call "Add State to Queue.vi"("State(s) In (\"\")"="idle" ("State(s) In (\"\")")) -> ("States Out"=w201:string)  [unwired: 14 in]
          }
          event "ORP偏移修正值": Value Change {
            n112 = event-data() -> ("NewVal"=w205:dbl)  [unwired: 1 in, 5 out]
            n113 = global read "多参数全局变量.vi" "MB session in"() -> (w207:refnum<class "MB_Master.lvclass">)
            n114 = call "000CH_ORP_ORP偏移修正值写入.vi"("数值"=w205, "MB session in"=w207) -> ("error out"=w206:errorcluster)  [unwired: 8 in, 1 out]
            n115 = call "Add State to Queue.vi"("State(s) In (\"\")"=w211, "State(s) At Back (\"\")"="idle" ("State(s) In (\"\")")) -> ("States Out"=w210:string)  [unwired: 13 in]
          }
          event "滤波设定": Value Change {
            n116 = event-data() -> ("NewVal"=w213:dbl)  [unwired: 1 in, 5 out]
            n117 = global read "多参数全局变量.vi" "MB session in"() -> (w214:refnum<class "MB_Master.lvclass">)
            n118 = call "0027H_ORP_数位滤波设定写入.vi"("数值"=w213, "MB session in"=w214) -> ("error out"=w212:errorcluster)  [unwired: 8 in, 1 out]
            n119 = call "Add State to Queue.vi"("State(s) In (\"\")"=w218, "State(s) At Back (\"\")"="idle" ("State(s) In (\"\")")) -> ("States Out"=w217:string)  [unwired: 13 in]
          }
          event "校准启动": Value Change {
            n120 = event-data() -> ()  [unwired: 1 in, 6 out]
            n121 = global read "多参数全局变量.vi" "校准运行状态"() -> (w220:T5)
            n122 = call "Add State to Queue.vi"("State(s) In (\"\")"=w225, "State(s) At Back (\"\")"="init: all\nCal: Place standard solution\n Cal: Calibration process\nidle" ("State(s) In (\"\")")) -> ("States Out"=w224:string)  [unwired: 13 in]
            n123 = Bundle By Name(cluster=w220, "ORP"=TRUE) -> (w221:T5)
            n124 = global write "多参数全局变量.vi" "校准运行状态"(w221) -> ()
          }
          event "校准停止": Value Change {
            n125 = event-data() -> ()  [unwired: 1 in, 6 out]
            n126 = call "Add State to Queue.vi"("State(s) In (\"\")"="init: all\nCal: Over\nidle" ("State(s) In (\"\")")) -> ("States Out"=w227:string)  [unwired: 14 in]
          }
          event "刷新按钮": Value Change {
            n127 = event-data() -> ()  [unwired: 1 in, 6 out]
            n128 = Two Button Dialog(message="请再次确实是否恢复出厂设置！" ("消息")) -> (T button?=w233:bool)  [unwired: 2 in]
            n129 = case shown="真" w233 {
              frame False {
              }
              frame True {
                w234 = u16 33 items=["Factory Reset"=33] ("数值")
                n130 = global read "多参数全局变量.vi" "MB session in"() -> (w235:refnum<class "MB_Master.lvclass">)
                n131 = call "0026H_ORP_命令寄存器写入.vi"("数值"=w234, "MB session in"=w235) -> ()  [unwired: 8 in, 2 out]
              }
            }
            n132 = call "Add State to Queue.vi"("State(s) In (\"\")"="init: all\nidle" ("State(s) In (\"\")")) -> ("States Out"=w230:string)  [unwired: 14 in]
          }
        }
      }
    }
  }
  n133 = while {
    stop <- FALSE stop-if-true
    n134 = global read "多参数全局变量.vi" "权限"() -> (w239:enum16{"一级权限", "二级权限", "三级权限"})
    n135 = Wait (ms)(milliseconds to wait=u32 1000 ("等待时间（毫秒）")) -> ()  [unwired: 1 out]
    n136 = Not Equal?(x=w239, y=enum16{"一级权限", "二级权限", "三级权限"}."一级权限") -> (x != y?=w236:bool)
    n137 = property on="滤波设定" class="DigNum (严格)"("Visible"=w236) -> ()  [unwired: 2 in, 2 out]
    n138 = property on="ORP偏移修正值" class="DigNum (严格)"("Visible"=w236) -> ()  [unwired: 2 in, 2 out]
  }
